vi "CHROMA Send Receive.vi"(8 "error in (no error)":errorcluster, 10 "Send Command":string, 11 "CHROMA VISA In":refnum<visa-resource-name>) -> (0 "error out":errorcluster, 2 "read buffer":string, 3 "CHROMA VISA Out":refnum<visa-resource-name>)   [LabVIEW 2020]
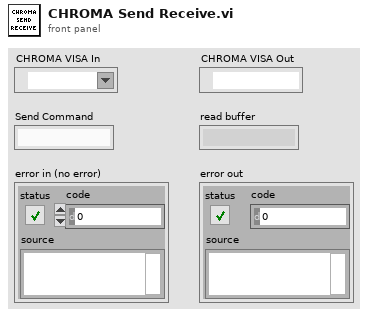
[diagram p1: front panel]
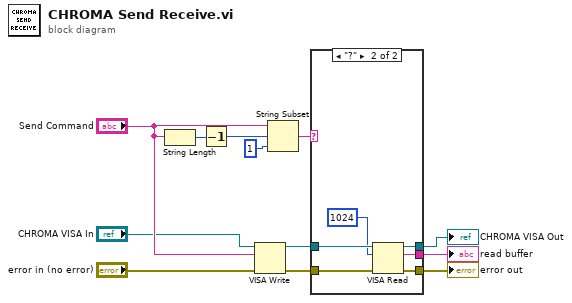
[diagram p0: block diagram]
diagram:
  n1 = String Length(string="Send Command") -> (length=w9:i32)
  n2 = Decrement(x=w9) -> (x-1=w8:i32)
  n3 = VISA Write(VISA resource name="CHROMA VISA In", write buffer="Send Command", error in (no error)="error in (no error)") -> (VISA resource name out=w1:refnum<visa-resource-name>, error out=w3:errorcluster)  [unwired: 1 out]
  n4 = String Subset(string="Send Command", offset (0)=w8, length (rest)=1 ("length (rest)")) -> (substring=w6:string)
  n5 = case shown="\"?\"" w6 {
    tunnel: w1 -> [w14 w20]
    tunnel: [w14 w19] -> w2
    tunnel: w3 -> [w13 w18]
    tunnel: [w13 w17] -> w11
    tunnel: [_ w15] -> w12
    frame "Not ?", Default {
    }
    frame "?" {
      n6 = VISA Read(VISA resource name=w20, byte count=u32 1024, error in (no error)=w18) -> (VISA resource name out=w19:refnum<visa-resource-name>, read buffer=w15:string, error out=w17:errorcluster)  [unwired: 1 out]
    }
  }
  "read buffer" <- w12
  "error out" <- w11
  "CHROMA VISA Out" <- w2
